vi "Write Single Coil.vi"(8 "error in (no error)":errorcluster, 9 "coil value":bool, 10 "address":u16, 11 "Modbus slave in":refnum<class "Modbus Master CR API.lvclass">) -> (0 "error out":errorcluster, 3 "Modbus slave out":refnum<class "Modbus Master CR API.lvclass">)   [LabVIEW 2021, in "Modbus Master CR API.lvclass"]
doc: "Writes a value to a single coil."
uses:
  Modbus Master CR API.lvclass
  Modbus Master CR API.lvclass/Modbus Master CR API.ctl
  Data Model/Device Data Model.lvclass
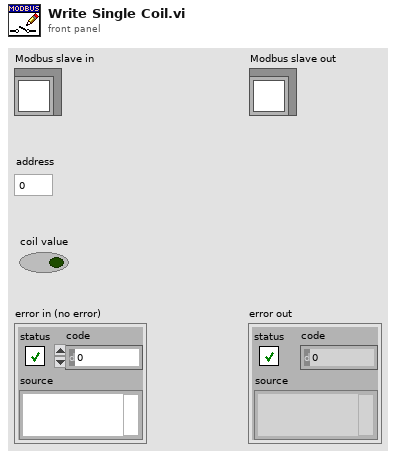
[diagram p1: front panel]
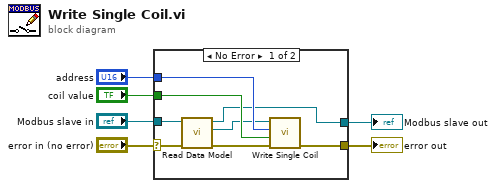
[diagram p0: block diagram]
diagram:
  n1 = case shown="No Error" "error in (no error)" {
    selector: "error in (no error)" -> [w11 w16]
    tunnel: [w12 w16] -> w5
    tunnel: "Modbus slave in" -> [w9 w15]
    tunnel: "coil value" -> [w14 _]
    tunnel: "address" -> [w13 _]
    tunnel: [w7 w15] -> w1
    frame No Error {
      n2 = call "Read Data Model.vi"("error in (no error)"=w11, "Modbus slave in"=w9) -> ("error out"=w10:errorcluster, "device data model"=w8:refnum<class "Device Data Model.lvclass">, "Modbus slave out"=w7:refnum<class "Modbus Master CR API.lvclass">)  [unwired: 7 in]
      n3 = call-dynamic "Write Single Coil.vi"("error in"=w10, "coil value"=w14, "address"=w13, "device data model in"=w8) -> ("error out"=w12:errorcluster)  [unwired: 6 in, 1 out]
    }
    frame Error {
    }
  }
  "error out" <- w5
  "Modbus slave out" <- w1
